vi "dscClearUserInterruptFunction.vi"(8 "error in":errorcluster, 11 "board":i16) -> (0 "error out":errorcluster, 3 "boardOut":i16)   [LabVIEW 2011, in "Diamond Universal Driver.lvlib"]
doc: "Use this template to build a dll driven application for the universal driver on Diamond PC/104 boards. This template sets up the VI for proper error handling and an entry point for the board. However, the <B>Call Library Function</B> node is not configured properly and must be configured by the user."
uses:
  Diamond Universal Driver.lvlib
  Controls/error codes.ctl
  Instruments/WL OPC/Support/dlls/dscud.dll
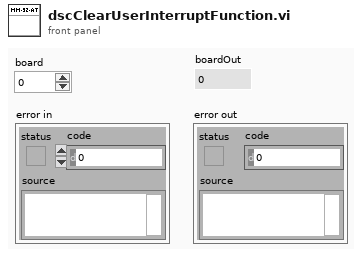
[diagram p1: front panel]
types:
  T1 = typedef "Diamond Universal Driver.lvlib/error codes.ctl" = enum8{"DE_NONE", "DE_HW_FAILURE", "DE_SW_FAILURE", "DE_HW_NOT_SUPPORTED", "DE_SW_NOT_SUPPORTED", "DE_INVALID_PARM", "DE_ALTERNATE_IN_PROGRESS", "DE_NONE_IN_PROGRESS", "DE_BUFFER_ROLLOVER", "DE_INVALID_ERROR_CODE", "DE_ALREADY_PAUSED", "DE_OVERFLOW", "DE_INVALID_FUNC", "DE_DSCUDH_INVALID", "DE_INVALID_BOARD", "DE_BOARD_LIMIT_REACHED", "DE_BOARD_BUSY", "DE_INVALID_WINDRVR_HANDLE", "DE_INVALID_WINDRVR_VERSION", "DE_BAD_WINDRVR_BOARD_INIT", "DE_OPERATION_TIMED_OUT", "DE_INVALID_WINDRVR_KP", "DE_THREAD_FAILURE"}
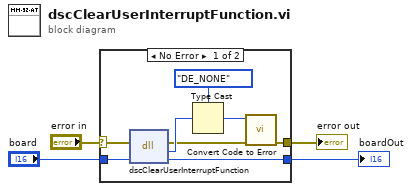
[diagram p0: block diagram]
diagram:
  n1 = case shown="No Error" "error in" {
    selector: "error in" -> [w12 w14]
    tunnel: [w8 w14] -> w3
    tunnel: [w6 w13] -> w2
    tunnel: "board" -> [w5 w13]
    frame No Error {
      n2 = dll-call lib="C:/Users/mrichardson/Documents/Web Based Version Control SW/Instruments/WL OPC/Support/dlls/dscud.dll" fn="dscClearUserInterruptFunction"(error in=w12, "board"=w5) -> (error out=w7:errorcluster, "error"=w11:u8, "board"=w6:i16)  [unwired: 2 in, 1 out]
      n3 = Type Cast(type=error_codes."DE_NONE" ("error codes"), x=w11) -> (*(type *) &x=w9:T1)
      n4 = call "Convert Code to Error.vi"("error in"=w7, "error codes"=w9) -> ("error out"=w8:errorcluster)  [unwired: 9 in]
    }
    frame Error {
    }
  }
  "error out" <- w3
  "boardOut" <- w2
